vi "Configure Limit Line Segment.vi"(0 "VISA resource name":refnum<visa-resource-name>, 1 "Stimulus Begin (0)":dbl, 2 "Response Begin (0)":dbl, 5 "Channel (1)":i32=1, 7 "Segment (1)":i32=1, 9 "Type of Limit Seg (2: OFF)":i32(ring)=2 items=["MIN", "MAX", "OFF"], 11 "error in (no error)":errorcluster, 12 "Stimulus End (0)":dbl, 13 "Response End (0)":dbl) -> (4 "VISA resource name out":refnum<visa-resource-name>, 15 "error out":errorcluster)   [LabVIEW 2018, in "Keysight PNA Series.lvlib"]
doc: "Configures a single limit line segment."
uses:
  Keysight PNA Series.lvlib
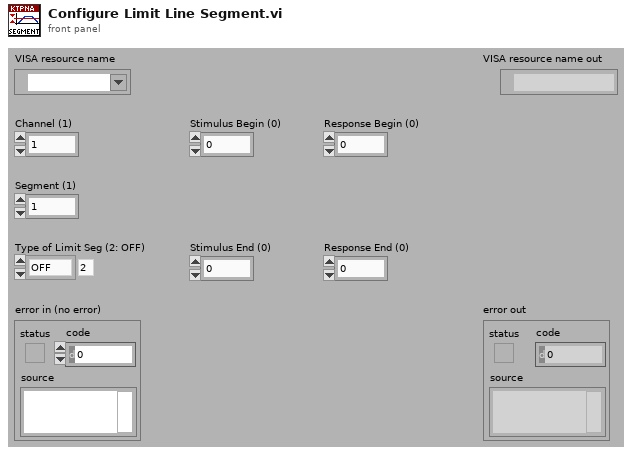
[diagram p1: front panel]
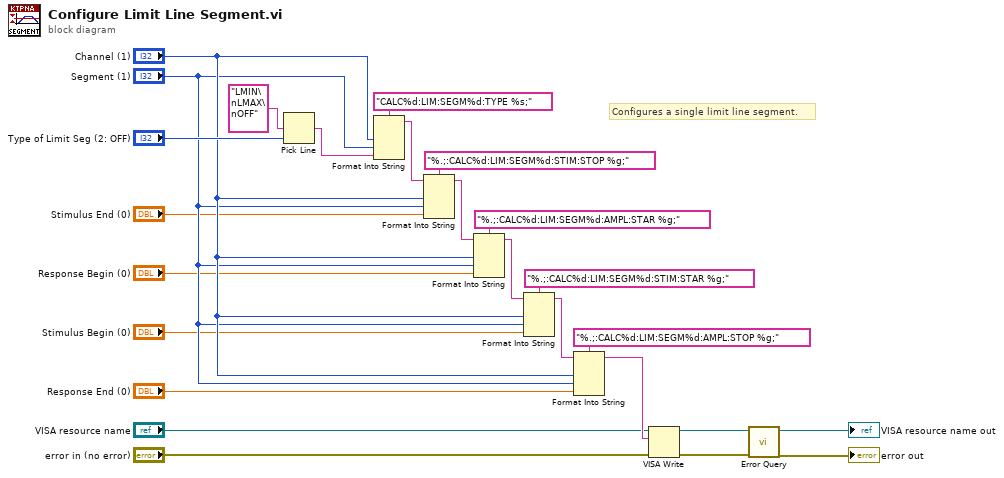
[diagram p0: block diagram]
diagram:
  # "Configures a single limit line segment."
  n1 = Pick Line(multi-line string="LMIN\nLMAX\nOFF", line index="Type of Limit Seg (2: OFF)") -> (output string=w20:string)  [unwired: 1 in]
  n2 = Format Into String(format string="CALC%d:LIM:SEGM%d:TYPE %s;", "Channel (1)", "Segment (1)", w20) -> (resulting string=w19:string)  [unwired: 2 in, 1 out]
  n3 = Format Into String(format string="%.;:CALC%d:LIM:SEGM%d:STIM:STOP %g;", initial string=w19, "Channel (1)", "Segment (1)", "Stimulus End (0)") -> (resulting string=w16:string)  [unwired: 1 in, 1 out]
  n4 = Format Into String(format string="%.;:CALC%d:LIM:SEGM%d:AMPL:STAR %g;", initial string=w16, "Channel (1)", "Segment (1)", "Response Begin (0)") -> (resulting string=w13:string)  [unwired: 1 in, 1 out]
  n5 = Format Into String(format string="%.;:CALC%d:LIM:SEGM%d:STIM:STAR %g;", initial string=w13, "Channel (1)", "Segment (1)", "Stimulus Begin (0)") -> (resulting string=w10:string)  [unwired: 1 in, 1 out]
  n6 = Format Into String(format string="%.;:CALC%d:LIM:SEGM%d:AMPL:STOP %g;", initial string=w10, "Channel (1)", "Segment (1)", "Response End (0)") -> (resulting string=w7:string)  [unwired: 1 in, 1 out]
  n7 = VISA Write(VISA resource name="VISA resource name", write buffer=w7, error in (no error)="error in (no error)") -> (VISA resource name out=w4:refnum<visa-resource-name>, error out=w3:errorcluster)  [unwired: 1 out]
  n8 = call "Error Query.vi"("error in (no error)"=w3, "VISA resource name"=w4) -> ("error out"=→"error out":errorcluster, "VISA resource name out"=→"VISA resource name out":refnum<visa-resource-name>)  [unwired: 6 in, 2 out]
